vi "ZCAN_InitCAN(EU).vi"(0 "device_hande":u32, 5 "can_index":u32, 7 "ZCAN_InitCAN_Setting_EU":T1, 11 "error in (no error)":errorcluster caption="错误输入（无错误）") -> (8 "can_index_handle":u32, 15 "error out":errorcluster caption="错误输出")   [LabVIEW 2018]
doc: "用于设置CAN通道的初始化参数。\n\n适用的设备：PCI-5010-U、PCI-5020-U、USBCAN-E-U、USBCAN-2E-U、CANalyst-II+"
uses:
  data_type/ZCAN_InitCAN_setting_EU.ctl
  bin/zlgcan_wrap.dll
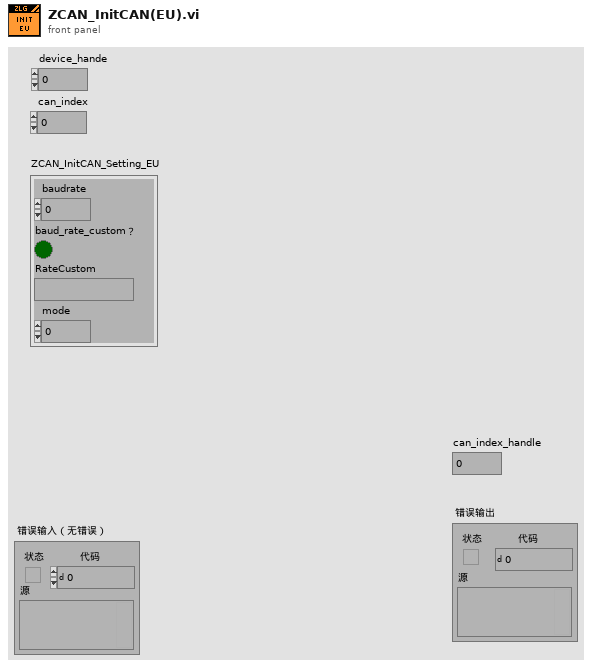
[diagram p1: front panel]
types:
  T1 = typedef "ZCAN_InitCAN_setting_EU.ctl" = cluster{"baudrate":u32, "baud_rate_custom？":bool, "RateCustom":string, "mode":u8}
  T2 = cluster{"can_type":u32, "can_type":u32, "can_type":u32, "can_type":u32, "can_type":u8, "can_type":u8, "can_type":u8, "mode":u8}
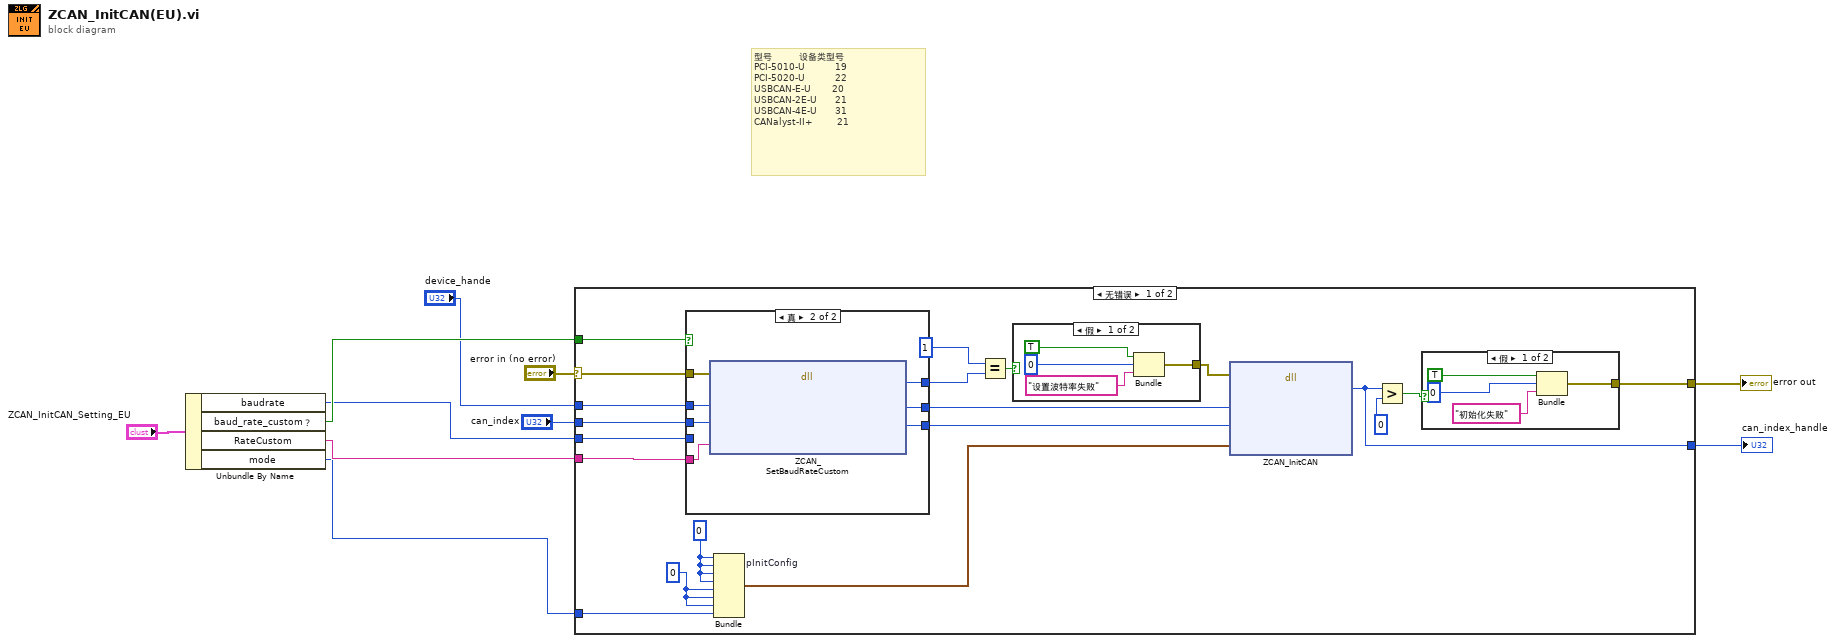
[diagram p0: block diagram]
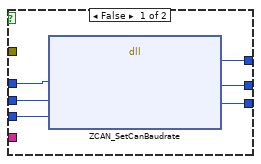
[diagram p4: hidden frame]
diagram:
  # "型号         设备类型号\nPCI-5010-U          19 \nPCI-5020-U          22\nUSBCAN-E-U       20\nUSBCAN-2E-U      21\nUSBCAN-4E-U      31\nCANalyst-II+        21"
  n1 = Unbundle By Name("ZCAN_InitCAN_Setting_EU") -> ("baudrate"=w3:u32, "baud_rate_custom？"=w5:bool, "RateCustom"=w2:string, "mode"=w1:u8)
  n2 = case shown="无错误" "error in (no error)" {
    selector: "error in (no error)" -> [w24 w52]
    tunnel: [w23 w52] -> w9
    tunnel: w5 -> [w30 _]
    tunnel: "device_hande" -> [w29 _]
    tunnel: "can_index" -> [w28 _]
    tunnel: w3 -> [w27 _]
    tunnel: w2 -> [w26 _]
    tunnel: w1 -> [w25 _]
    tunnel: [w22 _] -> w7
    frame No Error {
      w12 = u8 0 ("can_type")
      w13 = u32 0 ("can_type")
      n3 = case shown="真" w30 {
        tunnel: [w43 w51] -> w21
        tunnel: [w42 w50] -> w20
        tunnel: [w44 w49] -> w18
        tunnel: w29 -> [w41 w47]
        tunnel: w28 -> [w40 w46]
        tunnel: w27 -> [w39 _]
        tunnel: w26 -> [_ w48]
        tunnel: w24 -> [_ w45]
        frame False {
          n4 = dll-call lib="PTH2Fabs D\nUSBCANFD DEMO20200512USBCAN-I系列binzlgcan_wrap.dll" fn="ZCAN_SetCanBaudrate"("hDev"=w41, "can_index"=w40, "baudrate"=w39) -> ("return"=w44:u32, "hDev"=w43:u32, "can_index"=w42:u32)  [unwired: 4 in, 2 out]
        }
        frame True {
          n5 = dll-call lib="PTH2Fabs D\nUSBCANFD DEMO20200512USBCAN-I系列binzlgcan_wrap.dll" fn="ZCAN_SetBaudRateCustom"(error in=w45, "device_handle"=w47, "can_index"=w46, "RateCustom"=w48) -> ("return"=w49:u32, "device_handle"=w51:u32, "can_index"=w50:u32)  [unwired: 3 in, 2 out]
        }
      }
      n6 = Bundle "pInitConfig"("can_type"=w13, "can_type"=w13, "can_type"=w13, "can_type"=w13, "can_type"=w12, "can_type"=w12, "can_type"=w12, "mode"=w25) -> (w11:T2)  [unwired: 1 in]
      n7 = Equal?(x=1, y=w18) -> (x = y?=w17:bool)
      n8 = case shown="假" w17 {
        tunnel: [w35 _] -> w16
        frame False {
          n9 = Bundle("status"=TRUE, "code"=0, "消息"="设置波特率失败") -> (w35:cluster{"status":bool, "code":i32, "消息":string})  [unwired: 1 in]
        }
        frame True {
        }
      }
      n10 = dll-call lib="PTH2Fabs D\nUSBCANFD DEMO20200512USBCAN-I系列binzlgcan_wrap.dll" fn="ZCAN_InitCAN"(error in=w16, "device_handle"=w21, "can_index"=w20, "pInitConfig"=w11) -> ("can_handle"=w22:u32)  [unwired: 5 in, 2 out]
      n11 = Greater?(x=w22, y=0) -> (0:w14:bool)
      n12 = case shown="假" w14 {
        tunnel: [w31 _] -> w23
        frame False {
          n13 = Bundle("status"=TRUE, "code"=0, "消息"="初始化失败") -> (w31:cluster{"status":bool, "code":i32, "消息":string})  [unwired: 1 in]
        }
        frame True {
        }
      }
    }
    frame Error {
    }
  }
  "error out" <- w9
  "can_index_handle" <- w7
